vi "Find the Distance.vi"(11 "Relevant Data":T1[](array[typedef])) -> (3 "Distance":dbl)   [LabVIEW 2015]
uses:
  References/Relevant Data.ctl
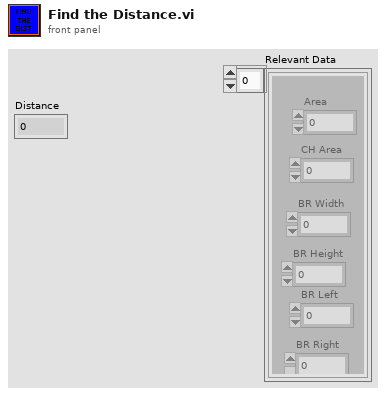
[diagram p1: front panel]
types:
  T1 = typedef "Relevant Data.ctl" = cluster{"Area":dbl, "CH Area":dbl, "BR Width":dbl, "BR Height":dbl, "BR Left":dbl, "BR Right":dbl}
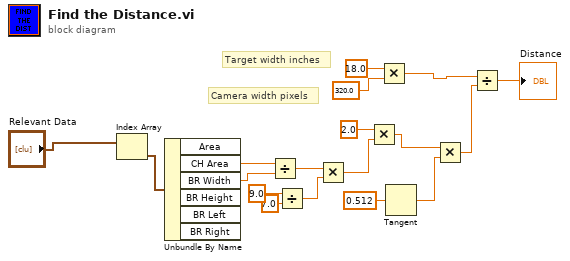
[diagram p0: block diagram]
diagram:
  # "Camera width pixels"
  # "Target width inches"
  n1 = Index Array(array="Relevant Data") -> (element=w17:T1)  [unwired: 1 in]
  n2 = Unbundle By Name(w17) -> ("CH Area"=w13:dbl, "BR Width"=w12:dbl)  [unwired: 4 out]
  n3 = Divide(x=w13, y=w12) -> (x/y=w11:dbl)
  n4 = Divide(x=9.0, y=7.0) -> (x/y=w10:dbl)
  n5 = Multiply(x=w11, y=w10) -> (x*y=w7:dbl)
  n6 = Multiply(x=2.0, y=w7) -> (x*y=w6:dbl)
  n7 = Multiply(x=18.0, y=320.0) -> (x*y=w1:dbl)
  n8 = Tangent(1:0.512 ("x")) -> (0:w4:dbl)
  n9 = Multiply(x=w6, y=w4) -> (x*y=w3:dbl)
  n10 = Divide(x=w1, y=w3) -> (x/y=→"Distance":dbl)
